vi "Begin.vi"(8 "error in":errorcluster) -> (0 "error out":errorcluster)   [LabVIEW 2015]
doc: "Called before other user functions, this VI is expected to open initial I/O refnums, load in file data, and do all program initialization. Notice that the <B>error out</B> terminal is simply used for data flow. Wiring it to other structures or subVIs ensures that this VI runs first."
uses:
  <vilib>/Rock Robotics/WPI/DriverStation/WPI_DriverStationRobotMode2.ctl
  <vilib>/Rock Robotics/SystemInterfaces/AI/FPGA_AIGyroChannel.ctl
  <vilib>/Rock Robotics/WPI/Accelerometer/WPI_AccelerometerRange.ctl
  <vilib>/Rock Robotics/WPI/Joystick/WPI_JoystickDeviceEnum.ctl
  <vilib>/Rock Robotics/WPI/CAN/TalonSRX/WPI_CANTalonSRX_APIControlMode.ctl
  <vilib>/Rock Robotics/WPI/CAN/TalonSRX/WPI_CANTalonSRX_BrakeOverride.ctl
  <vilib>/Rock Robotics/WPI/CAN/TalonSRX/WPI_CANTalonSRX_APIFeedbackSelect.ctl
  <vilib>/Rock Robotics/SystemInterfaces/i2clib/i2c_bus.ctl
  <vilib>/Rock Robotics/WPI/SerialPort/WPI_SerialPort.ctl
  <vilib>/Rock Robotics/WPI/Accelerometer/ADXL345 Range.ctl
  <vilib>/Rock Robotics/WPI/Accelerometer/WPI_AccelerometerADXL345 Axes.ctl
  <vilib>/Rock Robotics/SystemInterfaces/DIO/FPGA_DIOChannel.ctl
  <vilib>/Rock Robotics/SystemInterfaces/AI/FPGA_AIChannel.ctl
  <vilib>/Rock Robotics/SystemInterfaces/DIO/FPGA_DIOPWMChannel.ctl
  Robot Global Data.vi
  <vilib>/Rock Robotics/Network Tables/NT Write String Array.vi
  <vilib>/Rock Robotics/WPI/Utilities/WPI_GetSetVariantRefNum.vi
  <vilib>/Rock Robotics/WPI/Switch/WPI_SwitchOpenLimit.vi
  <vilib>/Rock Robotics/WPI/Accelerometer/WPI_AccelerometerADXL345_I2C_Open.vi
  <vilib>/Rock Robotics/WPI/MotorControl/WPI_MotorControlOpenCANTalonSRX.vi
  <vilib>/Rock Robotics/WPI/Accelerometer/InternalAccelerometer/WPI_AccelerometerInternalOpen.vi
  <vilib>/Rock Robotics/WPI/Gyro/WPI_GyroAnalogOpen.vi
panel:
  # "BEGIN.VI"
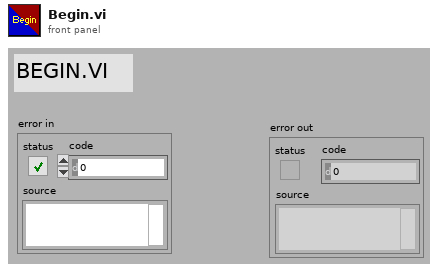
[diagram p1: front panel]
types:
  T1 = typedef "WPI_DriverStationRobotMode2.ctl" = enum16{"Autonomous Disabled", "Autonomous Enabled", "Teleop Disabled", "Teleop Enabled", "Disconnected", "Finish", "Test Disabled", "Test Enabled", "Emergency Stopped"}
  T2 = typedef "WPI_SerialPort.ctl" = enum16{"Onboard RS-232", "MXP TTL"}
  T3 = typedef "WPI_SerialPortRef.ctl" = cluster{"DevStatus":errorcluster, "Serial Port Name":refnum<visa-resource-name>}
  T4 = typedef "WPI_CANTalonSRX_APIFeedbackSelect.ctl" = enum16{"Digital Quadrature Encoder", "Analog Potentiometer", "Analog Encoder", "Count on Quad-A (Rising-Edge)", "Count on Quad-A (Falling-Edge)", "CTR Magnetic Enc (Absolute)", "CTR Magnetic Enc (Relative)", "Pulse Width"}
  T5 = typedef "WPI_CANTalonSRX_BrakeOverride.ctl" = enum8{"No Override", "Override to Coast", "Override to Brake"}
  T6 = typedef "WPI_CANTalonSRX_APIControlMode.ctl" = enum8{"Percent VBus", "Speed", "Position", "Slave", "Unchanged / Invalid", "Voltage Compensation", "Current", "Motion Profile"}
  T7 = typedef "WPI_MotorControlDeviceRef.ctl" = cluster{"DeviceStatus":errorcluster, "Type":T8, "PWM":cluster{"PWM Channel":T9, "DeadBand":T10}, "CAN":cluster{"Device Number":u8, "Control Mode":T11, "Semaphore":T12, "Max Vout":dbl, "TalonSRX Control Mode":T6}, "Invert":bool}
  T8 = typedef "WPI_MotorControlType.ctl" = enum16{"PWM", "CAN", "CANTalonSRX"}
  T9 = typedef "FPGA_DIOPWMChannel.ctl" = enum8{"PWM 0", "PWM 1", "PWM 2", "PWM 3", "PWM 4", "PWM 5", "PWM 6", "PWM 7", "PWM 8", "PWM 9", "PWM MXP 0", "PWM MXP 1", "PWM MXP 2", "PWM MXP 3", "PWM MXP 4", "PWM MXP 5", "PWM MXP 6", "PWM MXP 7", "PWM MXP 8", "PWM MXP 9", "Invalid"}
  T10 = typedef "WPI_PWMDeadband.ctl" = cluster{"Name":string, "maxPositivePwm":i32, "minPositivePwm":i32, "centerPwm":i32, "maxNegativePwm":i32, "minNegativePwm":i32, "angularRange":u16}
  T11 = typedef "WPI_CANJaguar_ControlMode.ctl" = enum8{"Percent VBus", "Current", "Speed", "Position", "Voltage"}
  T12 = typedef "Semaphore RefNum" = refnum<k1>
  T13 = typedef "WPI_CompressorDevRef.ctl" = cluster{"DevStatus":errorcluster, "Pneumatics Control Module":u8}
  T14 = typedef "WPI_JoystickDeviceEnum.ctl" = enum16{"USB 0", "USB 1", "USB 2", "USB 3", "USB 4", "USB 5"}
  T15 = typedef "WPI_JoystickDevRef.ctl" = cluster{"Device":T14}
  T16 = typedef "FPGA_AIChannel.ctl" = enum8{"AI 0", "AI 1", "AI 2", "AI 3", "AI MXP 0", "AI MXP 1", "AI MXP 2", "AI MXP 3", "Invalid"}
  T17 = typedef "WPI_AnalogChannelDevRef.ctl" = cluster{"DevStatus":errorcluster, "Analog Channel":T16}
  T18 = typedef "WPI_PotentiometerDevRef.ctl" = cluster{"DevStatus":errorcluster, "Analog Channel":T16, "Invert Output":bool}
  T19 = typedef "WPI_AccelerometerADXL345 Axes.ctl" = cluster{"X-Axis":bool, "Y-Axis":bool, "Z-Axis":bool}
  T20 = typedef "i2c_bus.ctl" = enum16{"I2C On-Board", "I2C MXP", "Invalid"}
  T21 = typedef "ADXL345 Range.ctl" = u8
  T22 = typedef "WPI_AccelerometerDevRef.ctl" = cluster{"DevStatus":errorcluster, "Scaling":T23, "Analog Channels":T24, "I2C Bus":T20, "SPI Bus":T25, "Accel Range":T21, "ADXL Axes":T19, "Handle":i32, "Device Address":u8, "Accel Type":enum16{"Analog", "ADXL345 I2C", "ADXL345 SPI", "Internal", "ADXL362 SPI"}}
  T23 = typedef "WPI_AccelerometerScaling.ctl" = cluster{"Gain (VoltsPerG)":dbl, "Center Voltage":dbl}
  T24 = typedef "WPI_AccelerometerAnalogChannels.ctl" = cluster{"X-Axis":T16, "Y-Axis":T16, "Z-Axis":T16}
  T25 = typedef "spi_bus.ctl" = enum16{"SPI On-Board, CS0", "SPI On-Board, CS1", "SPI On-Board, CS2", "SPI On-Board, CS3", "SPI MXP", "Invalid"}
  T26 = typedef "WPI_I2CDevRef.ctl" = cluster{"DevStatus":errorcluster, "Device Address":u8, "Handle":i32, "I2C Bus":T20}
  T27 = typedef "FPGA_DIOChannel.ctl" = enum8{"DIO 0", "DIO 1", "DIO 2", "DIO 3", "DIO 4", "DIO 5", "DIO 6", "DIO 7", "DIO 8", "DIO 9", "DIO MXP 0", "DIO MXP 1", "DIO MXP 2", "DIO MXP 3", "DIO MXP 4", "DIO MXP 5", "DIO MXP 6", "DIO MXP 7", "DIO MXP 8", "DIO MXP 9", "DIO MXP 10", "DIO MXP 11", "DIO MXP 12", "DIO MXP 13", "DIO MXP 14", "DIO MXP 15", "Invalid"}
  T28 = typedef "WPI_DigitalOutputDevRef.ctl" = cluster{"DIO Channel":T27, "DevStatus":errorcluster}
  T29 = typedef "WPI_SwitchDevRef.ctl" = cluster{"DevStatus":errorcluster, "DIO Channel":T27, "CntIndex":T30, "Normally Closed":bool}
  T30 = typedef "FPGA_CounterCtrSystemIndex.ctl" = enum8{"Ctr 0", "Ctr 1", "Ctr 2", "Ctr 3", "Ctr 4", "Ctr 5", "Ctr 6", "Ctr 7", "Invalid"}
  T31 = typedef "FPGA_AIGyroChannel.ctl" = enum8{"AI 0", "AI 1", "Invalid"}
  T32 = typedef "WPI_GyroDevRef.ctl" = cluster{"DevStatus":errorcluster, "Analog Channel":T16, "Offset":dbl, "Gain (VoltsPerDegree/Second)":dbl, "Gyro Type":enum16{"Analog", "XRS450"}, "Handle":i32, "SPI Bus":T25, "Device Found":bool, "Sample Rate":dbl, "Calibrate On Open":bool}
  T33 = typedef "WPI_ServoDeviceRef.ctl" = cluster{"DeviceStatus":errorcluster, "PWM Channel":T9, "DeadBand":T10}
  T34 = typedef "WPI_AccelerometerRange.ctl" = enum16{"+/- 2 g", "+/- 4 g", "+/- 8 g"}
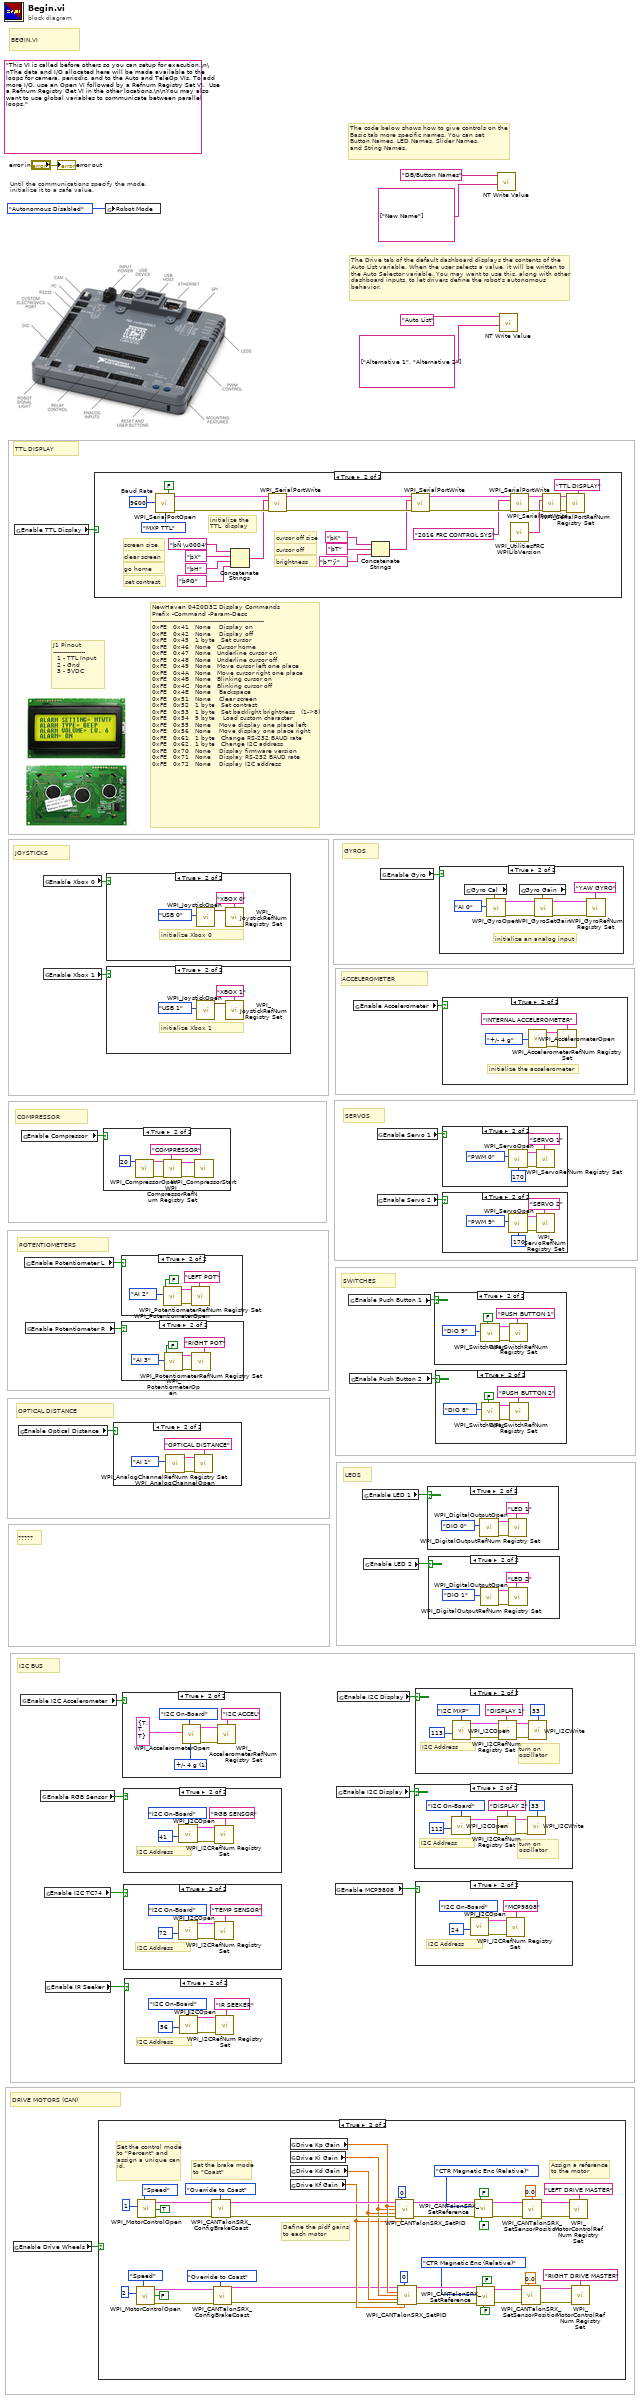
[diagram p0: block diagram]
diagram:
  (unwired) "This VI is called before others so you can setup for execution.\n\nThe data and I/O allocated here will be made available to the loops for camera, periodic, and to the Auto and TeleOp VIs. To add more I/O, use an Open VI followed by a Refnum Registry Set VI.  Use a Refnum Registry Get VI in the other locations.\n\nYou may also want to use global variables to communicate between parallel loops."
  # "GYROS"
  # "ACCELEROMETER"
  # "JOYSTICKS"
  # "DRIVE MOTORS (CAN)"
  # "I2C BUS"
  # "?????"
  # "LEDS"
  # "OPTICAL DISTANCE"
  # "SWITCHES"
  # "SERVOS"
  # "POTENTIOMETERS"
  # "COMPRESSOR"
  # "J1 Pinout\n----------------\n  1 - TTL Input\n  2 - Gnd\n  3 - 5VDC"
  # "NewHaven 0420D3Z Display Commands\nPrefix -Command -Param-Desc\n--------------------------------------------------------\n0xFE   0x41   None    Display on\n0xFE   0x42   None    Display off\n0xFE   0x45   1 byte   Set cursor\n0xFE   0x46   None   Cursor home\n0xFE   0x47   None   Underline cursor on\n0xFE   0x48   None   Underline cursor off\n0xFE   0x49   None   Move cursor left one place\n0xFE   0x4A   None   Move cursor right one place\n0xFE   0x4B   None   Blinking cursor on\n0xFE   0x4C   None   Blinking cursor off\n0xFE   0x4E   None    Backspace\n0xFE   0x51   None    Clear screen\n0xFE   0x52   1 byte   Set contrast\n0xFE   0x53   1 byte   Set backlight brightness   (1->8)\n0xFE   0x54   9 byte    Load custom character\n0xFE   0x55   None    Move display one place left\n0xFE   0x56   None    Move display one place right\n0xFE   0x61   1 byte   Change RS-232 BAUD rate\n0xFE   0x62   1 byte   Change I2C address\n0xFE   0x70   None    Display firmware version\n0xFE   0x71   None    Display RS-232 BAUD rate\n0xFE   0x72   None    Display I2C address"
  # "TTL DISPLAY"
  # "BEGIN.VI"
  # "The Drive tab of the default dashboard displays the contents of the\nAuto List variable. When the user selects a value, it will be written to\nthe Auto Selector variable. You may want to use this, along with other\ndashboard inputs, to let drivers define the robot's autonomous\nbehavior."
  # "The code below shows how to give controls on the\nBasic tab more specific names. You can set\nButton Names, LED Names, Slider Names,\nand String Names."
  # "Until the communications specify the mode,\ninitialize it to a safe value."
  n1 = global read "Robot Global Data.vi" "Enable Drive Wheels"() -> (w5:bool)
  n2 = global read "Robot Global Data.vi" "Enable TTL Display"() -> (w8:bool)
  n3 = global read "Robot Global Data.vi" "Enable Optical Distance"() -> (w16:bool)
  n4 = global read "Robot Global Data.vi" "Enable I2C Accelerometer"() -> (w12:bool)
  n5 = global read "Robot Global Data.vi" "Enable Compressor"() -> (w23:bool)
  n6 = global read "Robot Global Data.vi" "Enable Potentiometer L"() -> (w22:bool)
  n7 = global read "Robot Global Data.vi" "Enable Potentiometer R"() -> (w21:bool)
  n8 = global read "Robot Global Data.vi" "Enable RGB Sensor"() -> (w11:bool)
  n9 = global read "Robot Global Data.vi" "Enable Xbox 0"() -> (w3:bool)
  n10 = global read "Robot Global Data.vi" "Enable Xbox 1"() -> (w4:bool)
  n11 = global read "Robot Global Data.vi" "Enable I2C TC74"() -> (w9:bool)
  n12 = global read "Robot Global Data.vi" "Enable IR Seeker"() -> (w6:bool)
  n13 = case shown="True" w8 {
    frame False {
    }
    frame True {
      w52 = u32 9600  # Baud Rate
      # "brightness"
      # "cursor off"
      # "cursor off size"
      # "set contrast"
      # "go home"
      # "clear screen"
      # "screen size"
      # "initialize the\nTTL  display"
      n14 = call <vilib>:"WPI_SerialPortOpen.vi"("Baud Rate"=w52, "Enable Termination Char? (T)"=FALSE, "Serial Port"=WPI_SerialPort."MXP TTL") -> ("SerialPortRef"=w51:T3, "error out"=w50:errorcluster)  [unwired: 11 in]
      n15 = Concatenate Strings("þÑ \u0004" ("string"), "þX" ("string"), "þH" ("string"), "þPØ" ("string")) -> (w46:string)
      n16 = call <vilib>:"WPI_SerialPortWrite.vi"("error in (no error)"=w50, "Buffer"=w46, "SerialPortRef"=w51) -> ("error out"=w37:errorcluster, "SerialPortRef"=w38:T3)  [unwired: 6 in, 1 out]
      n17 = Concatenate Strings("þK" ("string"), "þT" ("string"), "þ™ÿ" ("string")) -> (w36:string)
      n18 = call <vilib>:"WPI_SerialPortWrite.vi"("error in (no error)"=w37, "Buffer"=w36, "SerialPortRef"=w38) -> ("error out"=w33:errorcluster, "SerialPortRef"=w35:T3)  [unwired: 6 in, 1 out]
      n19 = call <vilib>:"WPI_SerialPortWrite.vi"("error in (no error)"=w33, "Buffer"="2016 FRC CONTROL SYS", "SerialPortRef"=w35) -> ("error out"=w32:errorcluster, "SerialPortRef"=w34:T3)  [unwired: 6 in, 1 out]
      n20 = call <vilib>:"WPI_UtilitiesFRC WPILibVersion.vi"() -> ("Version"=w31:string)  [unwired: 14 in, 1 out]
      n21 = call <vilib>:"WPI_SerialPortWrite.vi"("error in (no error)"=w32, "Buffer"=w31, "SerialPortRef"=w34) -> ("error out"=w48:errorcluster, "SerialPortRef"=w49:T3)  [unwired: 6 in, 1 out]
      n22 = call <vilib>:"WPI_SerialPortRefNum Registry Set.vi"("error in (no error)"=w48, "refnum name"="TTL DISPLAY", "SerialPortRef"=w49) -> ()  [unwired: 7 in, 2 out]
    }
  }
  n23 = case shown="True" w5 {
    frame False {
    }
    frame True {
      # "Assign a reference to the motor"
      # "Set the brake mode to \"Coast\""
      # "Define the pidf gains to each motor"
      # "Set the control mode to \"Percent\" and assign a unique can id."
      n24 = call-poly <vilib>:"WPI_MotorControlOpen.vi"("Invert"=FALSE, "Device Number"=u8 2, "Control Mode"=WPI_CANTalonSRX_APIControlMode."Speed") -> ("error out"=w79:errorcluster, "MotorControlDeviceRef"=w80:T7)  [unwired: 7 in]
      n25 = call-poly <vilib>:"WPI_MotorControlOpen.vi"("Invert"=TRUE, "Device Number"=u8 1, "Control Mode"=WPI_CANTalonSRX_APIControlMode."Speed") -> ("error out"=w88:errorcluster, "MotorControlDeviceRef"=w87:T7)  [unwired: 7 in]
      n26 = call <vilib>:"WPI_CANTalonSRX_ConfigBrakeCoast.vi"("error in (no error)"=w88, "Brake / Coast Mode"=WPI_CANTalonSRX_BrakeOverride."Override to Coast", "CAN Talon SRX Ref"=w87) -> ("error out"=w93:errorcluster, "CAN Talon SRX Ref"=w94:T7)  [unwired: 7 in]
      n27 = call <vilib>:"WPI_CANTalonSRX_ConfigBrakeCoast.vi"("error in (no error)"=w79, "Brake / Coast Mode"=WPI_CANTalonSRX_BrakeOverride."Override to Coast", "CAN Talon SRX Ref"=w80) -> ("error out"=w81:errorcluster, "CAN Talon SRX Ref"=w82:T7)  [unwired: 7 in]
      n28 = global read "Robot Global Data.vi" "Drive Kp Gain"() -> (w92:dbl)
      n29 = global read "Robot Global Data.vi" "Drive Ki Gain"() -> (w91:dbl)
      n30 = global read "Robot Global Data.vi" "Drive Kd Gain"() -> (w90:dbl)
      n31 = global read "Robot Global Data.vi" "Drive Kf Gain"() -> (w89:dbl)
      n32 = call <vilib>:"WPI_CANTalonSRX_SetPID.vi"("CAN Talon SRX Ref"=w94, "Parameter Slot"=u8 0, "P"=w92, "I"=w91, "D"=w90, "error in (no error)"=w93, "F"=w89) -> ("CAN Talon SRX Ref"=w73:T7, "error out"=w75:errorcluster)  [unwired: 7 in]
      n33 = call <vilib>:"WPI_CANTalonSRX_SetPID.vi"("CAN Talon SRX Ref"=w82, "Parameter Slot"=u8 0, "P"=w92, "I"=w91, "D"=w90, "error in (no error)"=w81, "F"=w89) -> ("CAN Talon SRX Ref"=w61:T7, "error out"=w58:errorcluster)  [unwired: 7 in]
      n34 = call <vilib>:"WPI_CANTalonSRX_SetReference.vi"("Reverse Closed-Loop Output"=FALSE, "error in (no error)"=w75, "Reverse Feedback Sensor"=FALSE, "Feedback Reference"=WPI_CANTalonSRX_APIFeedbackSelect."CTR Magnetic Enc (Relative)", "CAN Talon SRX Ref"=w73) -> ("error out"=w68:errorcluster, "CAN Talon SRX Ref"=w67:T7)  [unwired: 5 in]
      n35 = call <vilib>:"WPI_CANTalonSRX_SetReference.vi"("Reverse Closed-Loop Output"=FALSE, "error in (no error)"=w58, "Reverse Feedback Sensor"=FALSE, "Feedback Reference"=WPI_CANTalonSRX_APIFeedbackSelect."CTR Magnetic Enc (Relative)", "CAN Talon SRX Ref"=w61) -> ("error out"=w59:errorcluster, "CAN Talon SRX Ref"=w60:T7)  [unwired: 5 in]
      n36 = call <vilib>:"WPI_CANTalonSRX_SetSensorPosition.vi"("error in (no error)"=w59, "New Sensor Position"=0.0, "CAN Talon SRX Ref"=w60) -> ("error out"=w63:errorcluster, "CAN Talon SRX Ref"=w64:T7)  [unwired: 7 in]
      n37 = call <vilib>:"WPI_CANTalonSRX_SetSensorPosition.vi"("error in (no error)"=w68, "New Sensor Position"=0.0, "CAN Talon SRX Ref"=w67) -> ("error out"=w74:errorcluster, "CAN Talon SRX Ref"=w72:T7)  [unwired: 7 in]
      n38 = call <vilib>:"WPI_MotorControlRefNum Registry Set.vi"("error in (no error)"=w74, "refnum name"="LEFT DRIVE MASTER", "MotorControlDevRef"=w72) -> ()  [unwired: 7 in, 2 out]
      n39 = call <vilib>:"WPI_MotorControlRefNum Registry Set.vi"("error in (no error)"=w63, "refnum name"="RIGHT DRIVE MASTER", "MotorControlDevRef"=w64) -> ()  [unwired: 7 in, 2 out]
    }
  }
  n40 = case shown="True" w23 {
    frame False {
    }
    frame True {
      n41 = call <vilib>:"WPI_CompressorOpen.vi"("Pneumatics Control Module (0)"=u8 20) -> ("CompressorDevRef"=w103:T13, "error out"=w104:errorcluster)  [unwired: 13 in]
      n42 = call <vilib>:"WPI_CompressorRefNum Registry Set.vi"("error in (no error)"=w104, "refnum name"="COMPRESSOR", "CompressorDevRef"=w103) -> ("error out"=w100:errorcluster, "CompressorDevRef"=w99:T13)  [unwired: 7 in]
      n43 = call <vilib>:"WPI_CompressorStart.vi"("error in (no error)"=w100, "CompressorDevRef"=w99) -> ()  [unwired: 8 in, 2 out]
    }
  }
  n44 = global write "Robot Global Data.vi" "Robot Mode"(WPI_DriverStationRobotMode2."Autonomous Disabled" ("Robot Mode")) -> ()
  n45 = case shown="True" w3 {
    frame False {
    }
    frame True {
      # "initialize Xbox 0"
      n46 = call <vilib>:"WPI_JoystickOpen.vi"("JoystickDevice"=WPI_JoystickDeviceEnum."USB 0") -> ("JoystickDevRef"=w106:T15)  [unwired: 10 in]
      n47 = call <vilib>:"WPI_JoystickRefNum Registry Set.vi"("refnum name"="XBOX 0", "JoystickDevRef"=w106) -> ()  [unwired: 8 in, 2 out]
    }
  }
  n48 = case shown="True" w4 {
    frame False {
    }
    frame True {
      # "initialize Xbox 1"
      n49 = call <vilib>:"WPI_JoystickOpen.vi"("JoystickDevice"=WPI_JoystickDeviceEnum."USB 1") -> ("JoystickDevRef"=w109:T15)  [unwired: 10 in]
      n50 = call <vilib>:"WPI_JoystickRefNum Registry Set.vi"("refnum name"="XBOX 1", "JoystickDevRef"=w109) -> ()  [unwired: 8 in, 2 out]
    }
  }
  n51 = case shown="True" w16 {
    frame False {
    }
    frame True {
      n52 = call <vilib>:"WPI_AnalogChannelOpen.vi"("Analog Channel"=FPGA_AIChannel."AI 1") -> ("error out"=w114:errorcluster, "AIDeviceRef"=w113:T17)  [unwired: 9 in]
      n53 = call <vilib>:"WPI_AnalogChannelRefNum Registry Set.vi"("error in (no error)"=w114, "refnum name"="OPTICAL DISTANCE", "AIDeviceRef"=w113) -> ()  [unwired: 7 in, 2 out]
    }
  }
  n54 = case shown="True" w22 {
    frame False {
    }
    frame True {
      n55 = call <vilib>:"WPI_PotentiometerOpen.vi"("Invert Output"=FALSE, "Analog Channel"=FPGA_AIChannel."AI 2") -> ("error out"=w119:errorcluster, "PotDevRef"=w118:T18)  [unwired: 8 in]
      n56 = call <vilib>:"WPI_PotentiometerRefNum Registry Set.vi"("error in (no error)"=w119, "refnum name"="LEFT POT", "PotDevRef"=w118) -> ()  [unwired: 7 in, 2 out]
    }
  }
  n57 = case shown="True" w21 {
    frame False {
    }
    frame True {
      n58 = call <vilib>:"WPI_PotentiometerOpen.vi"("Invert Output"=FALSE, "Analog Channel"=FPGA_AIChannel."AI 3") -> ("error out"=w124:errorcluster, "PotDevRef"=w123:T18)  [unwired: 8 in]
      n59 = call <vilib>:"WPI_PotentiometerRefNum Registry Set.vi"("error in (no error)"=w124, "refnum name"="RIGHT POT", "PotDevRef"=w123) -> ()  [unwired: 7 in, 2 out]
    }
  }
  n60 = case shown="True" w12 {
    frame False {
    }
    frame True {
      w129 = T21 1 items=["+/- 2 g", "+/- 4 g", "+/- 8 g", "+/- 16 g"] ("Accel Range")
      n61 = call-poly <vilib>:"WPI_AccelerometerOpen.vi"("I2C Bus"=i2c_bus."I2C On-Board", "Accel Range"=w129, "ADXL345 Axes"=T19 {"X-Axis"=TRUE, "Y-Axis"=TRUE, "Z-Axis"=TRUE}) -> ("error out"=w127:errorcluster, "AccelerometerDevRef"=w126:T22)  [unwired: 7 in]
      n62 = call <vilib>:"WPI_AccelerometerRefNum Registry Set.vi"("error in (no error)"=w127, "refnum name"="I2C ACCEL", "AccelerometerDevRef"=w126) -> ()  [unwired: 7 in, 2 out]
    }
  }
  n63 = case shown="True" w11 {
    frame False {
    }
    frame True {
      # "I2C Address"
      n64 = call <vilib>:"WPI_I2COpen.vi"("Device Address"=u8 41, "I2C Bus"=i2c_bus."I2C On-Board") -> ("error out"=w133:errorcluster, "I2CDevRef"=w132:T26)  [unwired: 8 in]
      n65 = call <vilib>:"WPI_I2CRefNum Registry Set.vi"("error in (no error)"=w133, "refnum name"="RGB SENSOR", "I2CDevRef"=w132) -> ()  [unwired: 7 in, 2 out]
    }
  }
  n66 = case shown="True" w9 {
    frame False {
    }
    frame True {
      # "I2C Address"
      n67 = call <vilib>:"WPI_I2COpen.vi"("Device Address"=u8 72, "I2C Bus"=i2c_bus."I2C On-Board") -> ("error out"=w138:errorcluster, "I2CDevRef"=w137:T26)  [unwired: 8 in]
      n68 = call <vilib>:"WPI_I2CRefNum Registry Set.vi"("error in (no error)"=w138, "refnum name"="TEMP SENSOR", "I2CDevRef"=w137) -> ()  [unwired: 7 in, 2 out]
    }
  }
  n69 = case shown="True" w6 {
    frame False {
    }
    frame True {
      # "I2C Address"
      n70 = call <vilib>:"WPI_I2COpen.vi"("Device Address"=u8 56, "I2C Bus"=i2c_bus."I2C On-Board") -> ("error out"=w143:errorcluster, "I2CDevRef"=w142:T26)  [unwired: 8 in]
      n71 = call <vilib>:"WPI_I2CRefNum Registry Set.vi"("error in (no error)"=w143, "refnum name"="IR SEEKER", "I2CDevRef"=w142) -> ()  [unwired: 7 in, 2 out]
    }
  }
  n72 = global read "Robot Global Data.vi" "Enable MCP9808"() -> (w7:bool)
  n73 = global read "Robot Global Data.vi" "Enable I2C Display"() -> (w10:bool)
  n74 = global read "Robot Global Data.vi" "Enable I2C Display"() -> (w13:bool)
  n75 = global read "Robot Global Data.vi" "Enable Push Button 1"() -> (w18:bool)
  n76 = global read "Robot Global Data.vi" "Enable Push Button 2"() -> (w17:bool)
  n77 = global read "Robot Global Data.vi" "Enable Accelerometer"() -> (w2:bool)
  n78 = global read "Robot Global Data.vi" "Enable LED 1"() -> (w15:bool)
  n79 = global read "Robot Global Data.vi" "Enable LED 2"() -> (w14:bool)
  n80 = global read "Robot Global Data.vi" "Enable Servo 1"() -> (w20:bool)
  n81 = global read "Robot Global Data.vi" "Enable Servo 2"() -> (w19:bool)
  n82 = global read "Robot Global Data.vi" "Enable Gyro"() -> (w1:bool)
  n83 = case shown="True" w10 {
    frame False {
    }
    frame True {
      # "I2C Address"
      # "turn on oscillator"
      n84 = call <vilib>:"WPI_I2COpen.vi"("Device Address"=u8 112, "I2C Bus"=i2c_bus."I2C On-Board") -> ("error out"=w146:errorcluster, "I2CDevRef"=w147:T26)  [unwired: 8 in]
      n85 = call <vilib>:"WPI_I2CRefNum Registry Set.vi"("error in (no error)"=w146, "refnum name"="DISPLAY 2", "I2CDevRef"=w147) -> ("error out"=w151:errorcluster, "I2CDevRef"=w152:T26)  [unwired: 7 in]
      n86 = call <vilib>:"WPI_I2CWrite.vi"("error in (no error)"=w151, "I2CRegister"=u8 33, "I2CDevRef"=w152) -> ()  [unwired: 7 in, 2 out]
    }
  }
  n87 = case shown="True" w13 {
    frame False {
    }
    frame True {
      # "I2C Address"
      # "turn on oscillator"
      n88 = call <vilib>:"WPI_I2COpen.vi"("Device Address"=u8 113, "I2C Bus"=i2c_bus."I2C MXP") -> ("error out"=w154:errorcluster, "I2CDevRef"=w155:T26)  [unwired: 8 in]
      n89 = call <vilib>:"WPI_I2CRefNum Registry Set.vi"("error in (no error)"=w154, "refnum name"="DISPLAY 1", "I2CDevRef"=w155) -> ("error out"=w159:errorcluster, "I2CDevRef"=w160:T26)  [unwired: 7 in]
      n90 = call <vilib>:"WPI_I2CWrite.vi"("error in (no error)"=w159, "I2CRegister"=u8 33, "I2CDevRef"=w160) -> ()  [unwired: 7 in, 2 out]
    }
  }
  n91 = case shown="True" w7 {
    frame False {
    }
    frame True {
      # "I2C Address"
      n92 = call <vilib>:"WPI_I2COpen.vi"("Device Address"=u8 24, "I2C Bus"=i2c_bus."I2C On-Board") -> ("error out"=w164:errorcluster, "I2CDevRef"=w163:T26)  [unwired: 8 in]
      n93 = call <vilib>:"WPI_I2CRefNum Registry Set.vi"("error in (no error)"=w164, "refnum name"="MCP9808", "I2CDevRef"=w163) -> ()  [unwired: 7 in, 2 out]
    }
  }
  n94 = case shown="True" w15 {
    frame False {
    }
    frame True {
      n95 = call <vilib>:"WPI_DigitalOutputOpen.vi"("DIO Channel"=FPGA_DIOChannel."DIO 0") -> ("error out"=w170:errorcluster, "DigitalOutputDevRef"=w167:T28)  [unwired: 9 in]
      n96 = call <vilib>:"WPI_DigitalOutputRefNum Registry Set.vi"("error in (no error)"=w170, "refnum name"="LED 1", "DigitalOutputDevRef"=w167) -> ()  [unwired: 7 in, 2 out]
    }
  }
  n97 = case shown="True" w14 {
    frame False {
    }
    frame True {
      n98 = call <vilib>:"WPI_DigitalOutputOpen.vi"("DIO Channel"=FPGA_DIOChannel."DIO 1") -> ("error out"=w174:errorcluster, "DigitalOutputDevRef"=w171:T28)  [unwired: 9 in]
      n99 = call <vilib>:"WPI_DigitalOutputRefNum Registry Set.vi"("error in (no error)"=w174, "refnum name"="LED 2", "DigitalOutputDevRef"=w171) -> ()  [unwired: 7 in, 2 out]
    }
  }
  n100 = case shown="True" w18 {
    frame False {
    }
    frame True {
      n101 = call-poly <vilib>:"WPI_SwitchOpen.vi"("Normally Closed"=FALSE, "DIO Channel"=FPGA_DIOChannel."DIO 9") -> ("error out"=w179:errorcluster, "SwitchDevRef"=w178:T29)  [unwired: 8 in]
      n102 = call <vilib>:"WPI_SwitchRefNum Registry Set.vi"("error in (no error)"=w179, "refnum name"="PUSH BUTTON 1", "SwitchDevRef"=w178) -> ()  [unwired: 7 in, 2 out]
    }
  }
  n103 = case shown="True" w17 {
    frame False {
    }
    frame True {
      n104 = call-poly <vilib>:"WPI_SwitchOpen.vi"("Normally Closed"=FALSE, "DIO Channel"=FPGA_DIOChannel."DIO 8") -> ("error out"=w184:errorcluster, "SwitchDevRef"=w183:T29)  [unwired: 8 in]
      n105 = call <vilib>:"WPI_SwitchRefNum Registry Set.vi"("error in (no error)"=w184, "refnum name"="PUSH BUTTON 2", "SwitchDevRef"=w183) -> ()  [unwired: 7 in, 2 out]
    }
  }
  n106 = case shown="True" w1 {
    frame False {
    }
    frame True {
      # "initialize an analog input"
      n107 = global read "Robot Global Data.vi" "Gyro Cal"() -> (w185:dbl)
      n108 = call-poly <vilib>:"WPI_GyroOpen.vi"("Calibrated Center Voltage"=w185, "Analog Channel"=FPGA_AIGyroChannel."AI 0") -> ("error out"=w188:errorcluster, "GyroDevRef"=w190:T32)  [unwired: 7 in, 1 out]
      n109 = global read "Robot Global Data.vi" "Gyro Gain"() -> (w186:dbl)
      n110 = call <vilib>:"WPI_GyroSetGain.vi"("error in (no error)"=w188, "Gain (VoltsPerDegree/Second)"=w186, "GyroDevRef"=w190) -> ("error out"=w187:errorcluster, "GyroDevRef"=w189:T32)  [unwired: 7 in]
      n111 = call <vilib>:"WPI_GyroRefNum Registry Set.vi"("error in (no error)"=w187, "refnum name"="YAW GYRO", "GyroDevRef"=w189) -> ()  [unwired: 7 in, 2 out]
    }
  }
  n112 = case shown="True" w20 {
    frame False {
    }
    frame True {
      n113 = call <vilib>:"WPI_ServoOpen.vi"("Angular Range"=u16 170, "PWM Channel"=FPGA_DIOPWMChannel."PWM 0") -> ("error out"=w197:errorcluster, "ServoDeviceRef"=w195:T33)  [unwired: 8 in]
      n114 = call <vilib>:"WPI_ServoRefNum Registry Set.vi"("error in (no error)"=w197, "refnum name"="SERVO 1", "ServoDeviceRef"=w195) -> ()  [unwired: 7 in, 2 out]
    }
  }
  n115 = case shown="True" w2 {
    frame False {
    }
    frame True {
      # "initialize the accelerometer"
      n116 = call-poly <vilib>:"WPI_AccelerometerOpen.vi"("Accel Range"=WPI_AccelerometerRange."+/- 4 g") -> ("error out"=w200:errorcluster, "AccelerometerDevRef"=w201:T22)  [unwired: 9 in]
      n117 = call <vilib>:"WPI_AccelerometerRefNum Registry Set.vi"("error in (no error)"=w200, "refnum name"="INTERNAL ACCELEROMETER", "AccelerometerDevRef"=w201) -> ()  [unwired: 7 in, 2 out]
    }
  }
  n118 = case shown="True" w19 {
    frame False {
    }
    frame True {
      n119 = call <vilib>:"WPI_ServoOpen.vi"("Angular Range"=u16 170, "PWM Channel"=FPGA_DIOPWMChannel."PWM 9") -> ("error out"=w206:errorcluster, "ServoDeviceRef"=w204:T33)  [unwired: 8 in]
      n120 = call <vilib>:"WPI_ServoRefNum Registry Set.vi"("error in (no error)"=w206, "refnum name"="SERVO 2", "ServoDeviceRef"=w204) -> ()  [unwired: 7 in, 2 out]
    }
  }
  n121 = call-poly <vilib>:"NT Write Value.vi"("String Array"=string[] ["New Name"], "Name"="DB/Button Names") -> ()  [unwired: 9 in, 1 out]
  n122 = call-poly <vilib>:"NT Write Value.vi"("String Array"=string[] ["Alternative 1", "Alternative 2"], "Name"="Auto List") -> ()  [unwired: 9 in, 1 out]
  "error out" <- "error in"
